vi "test.ingest_journalJSON v2.vi"   [LabVIEW 2020]
uses:
  datasources/dataset/dataset.lvclass
  nominal types/channelConfig/channelConfig.lvclass
  Nominal Client/Nominal Client.lvclass/Nominal Client.ctl
  nominal types/workspace/workspace.lvclass/workspace.ctl
  f68fde30-30e4-4b08-97bf-6f7da0132bc9.vi
  d999190f-fee9-49b3-afb9-f232f2b660b8.vi
  Nominal Client/private_data.set.vi
  nominal types/workspace/rid.get.vi
  nominal types/workspace/id.get.vi
  <vilib>/AdvancedString/1D String Array to Delimited String.vi
  Nominal Client/workspace.set.vi
  datasources/s3/s3.lvclass
  C:/code/labview-client/lv_src/datasources/source/source.lvclass
  <vilib>/Utility/error.llb/Error Cluster From Error Code.vi
  Nominal Client/Palette Items/who_am_i.vi
  Nominal Client/workspace_cache.get_from_rid.vi
  Nominal Client/workspace_cache.get.vi
  datasources/target/create_new.vi
  datasources/source/create_s3.vi
  Nominal Client/ingest_journalJson.vi
  User/User.lvclass
  Nominal Client/Nominal Client.lvclass
  nominal types/workspace/workspace.lvclass
  submodules/reqwest-labview/lv-src/reqwest/reqwest.lvclass
  datasources/source/source.lvclass
  datasources/target/target.lvclass
  nominal types/properties/properties.lvclass
  C:/code/labview-client/lv_src/datasources/payload/payload.lvclass
  C:/code/labview-client/lv_src/datasources/s3/s3.lvclass
types:
  T1 = cluster{"dataset":refnum<class "dataset.lvclass">, "channelConfig":refnum<class "channelConfig.lvclass">}
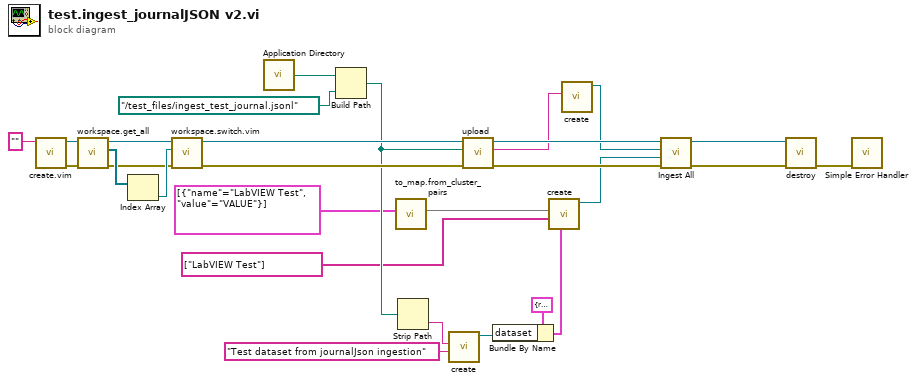
[diagram p0: block diagram]
diagram:
  n1 = call "create.vim"("API Token (string or path)"="") -> ("error out"=w14:errorcluster, "Nominal Client"=w18:refnum<class "Nominal Client.lvclass">)  [unwired: 8 in, 1 out]
  n2 = call "workspace.get_all.vi"("error in"=w14, "Nominal Client in"=w18) -> ("error out"=w13:errorcluster, "Workspaces"=w16:refnum<class "workspace.lvclass">[], "Nominal Client out"=w17:refnum<class "Nominal Client.lvclass">)  [unwired: 7 in]
  n3 = Index Array(array=w16) -> (element=w15:refnum<class "workspace.lvclass">)  [unwired: 1 in]
  n4 = call "workspace.switch.vim"("error in"=w13, "Workspace (Object, RID, Path)"=w15, "Nominal Client in"=w17) -> ("error out"=w12:errorcluster, "Nominal Client out"=w11:refnum<class "Nominal Client.lvclass">)  [unwired: 7 in]
  n5 = call <vilib>:"Application Directory.vi"() -> ("Application Directory"=w20:path)
  n6 = Build Path(base path=w20, name or relative path=path "../test_files/ingest_test_journal.jsonl") -> (appended path=w6:path)
  n7 = call "to_map.from_cluster_pairs.vi"("properties (cluster pairs)"=cluster{"name":string, "value":string}[] [{"name"="LabVIEW Test", "value"="VALUE"}] ("properties")) -> ("properties (map)"=w1:map{string, string})  [unwired: 10 in]
  n8 = Strip Path(path=w6) -> (name=w5:string)  [unwired: 1 out]
  n9 = call "create.vi"("Description"="Test dataset from journalJson ingestion", "Name"=w5) -> ("dataset"=w8:refnum<class "dataset.lvclass">)  [unwired: 9 in]
  n10 = call "upload.vi"("error in"=w12, "File"=w6, "Nominal Client in"=w11) -> ("error out"=w25:errorcluster, "Path to S3 File"=w24:string, "Nominal Client out"=w26:refnum<class "Nominal Client.lvclass">)  [unwired: 6 in]
  n11 = Bundle By Name(cluster=T1 {"dataset"=refnum, "channelConfig"=refnum} ("Optional"), "dataset"=w8) -> (w9:T1)
  n12 = call-poly "create.vi"("Optional"=w9, "Labels"=string[] ["LabVIEW Test"] ("labels"), "Properties"=w1) -> ("New Target"=w22:refnum<class "target.lvclass">)  [unwired: 8 in]
  n13 = call-poly "create.vi"("Path"=w24) -> ("source"=w23:refnum<class "s3.lvclass">)  [unwired: 10 in]
  n14 = call-poly "Ingest All.vi"("error in"=w25, "Target"=w22, "Source"=w23, "Nominal Client in"=w26) -> ("error out"=w27:errorcluster, "Nominal Client out"=w28:refnum<class "Nominal Client.lvclass">)  [unwired: 4 in, 2 out]
  n15 = call "destroy.vi"("error in"=w27, "Nominal Client"=w28) -> ("error out"=w4:errorcluster)  [unwired: 9 in]
  n16 = call <vilib>:"Simple Error Handler.vi"("error in (no error)"=w4) -> ()  [unwired: 4 in, 5 out]
